vi "Process Monitor Test.vi"() -> ()   [LabVIEW 2018]
uses:
  Core/Assert API Components/Assert API Components.lvlib
panel:
  out "Numeric":i32
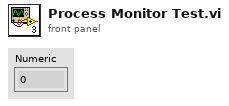
[diagram p1: front panel]
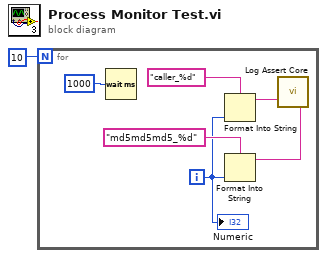
[diagram p0: block diagram]
diagram:
  n1 = for {
    N: 10 -> [_]
    i -> [w3]
    n2 = Wait (ms)(milliseconds to wait=u32 1000) -> ()  [unwired: 1 out]
    n3 = Format Into String(format string="caller_%d" ("Calling VI Name"), w3) -> (resulting string=w6:string)  [unwired: 2 in, 1 out]
    n4 = Format Into String(format string="md5md5md5_%d" ("MD5"), w3) -> (resulting string=w4:string)  [unwired: 2 in, 1 out]
    n5 = call "Log Assert Core.vi"("Calling VI Name"=w6, "MD5"=w4) -> ()  [unwired: 18 in]
    "Numeric" <- w3
  }
